vi "Include_when_Saving.vi"(8 "error in (no error)":errorcluster, 11 "AB_Source_Container in":refnum<class "AB_Source_Container.lvclass">) -> (0 "error out":errorcluster, 2 "include":bool, 3 "AB_Source_Container out":refnum<class "AB_Source_Container.lvclass">)   [LabVIEW 2020, in "AB_Source_Container.lvclass"]
uses:
  <vilib>/AppBuilder/AB_Classes/Source/Container/AB_Source_Container.lvclass
  e:/builds/penguin/labview/branches/2020/dev/dist/vi.lib/AppBuilder/AB_Classes/Source/AB_Source.lvclass
  <vilib>/AppBuilder/AB_Classes/Source/Container/AB_Source_Container.lvclass/AB_Source_Container.ctl
  <vilib>/AppBuilder/AB_Classes/Source/AB_Source.lvclass
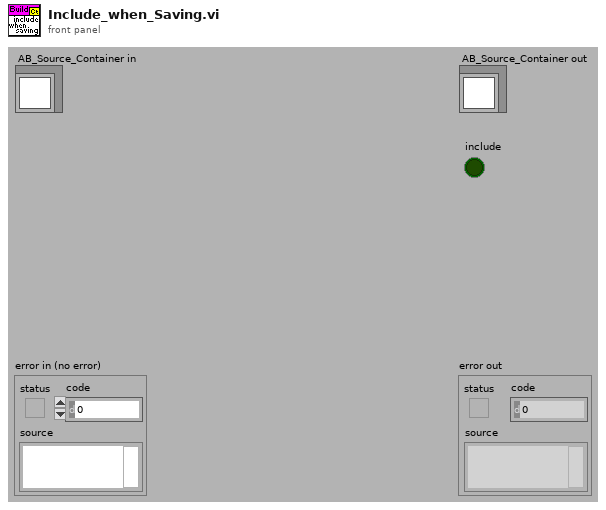
[diagram p1: front panel]
types:
  T1 = typedef "AB_Source.ctl" = cluster{"path":path, "itemID":string, "parentIndex":i32, "sourceInclusion":T2, "destinationIndex":i32, "properties":T3[], "newName":string, "lvfile":bool, "valid":bool, "eng_inBuild":bool, "eng_isNonVILink":bool, "Amalgamation":bool, "Amalgamation Piece":bool, "eng_delimitedName":string, "preventRename":bool}
  T2 = typedef "AB_Source_Inclusion.ctl" = enum16{"IncludeIfReferenced", "Include", "Exclude", "TopLevel"}
  T3 = typedef "AB_Source_Properties.ctl" = cluster{"sourcePropertyType":T4, "value":variant}
  T4 = typedef "AB_Source_Property_Type.ctl" = enum16{"Remove block diagram", "Remove front panel", "Password", "Window has title bar", "Show menu bar", "Show vertical scroll bar", "Show horizontal scroll bar", "Show toolbar", "Show Abort button", "Show fp when called", "Window behavior", "Allow user to close window", "Window run-time position", "Run when opened", "Allow debugging", "Auto error handling", "Generate guard code", "Use stack variables", "Expression folding", "Integer only", "Inline subVI"}
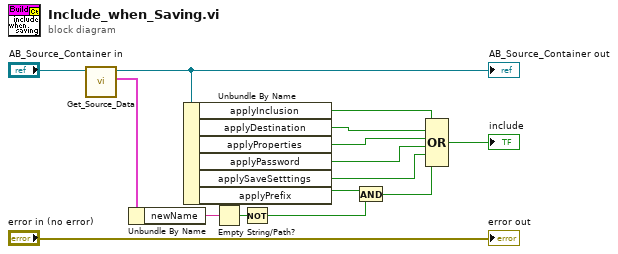
[diagram p0: block diagram]
diagram:
  n1 = call <vilib>:"Get_Source_Data.vi"("Class in"="AB_Source_Container in") -> ("data"=w2:T1, "Class out"=w3:refnum<class "AB_Source_Container.lvclass">)  [unwired: 8 in, 1 out]
  "AB_Source_Container out" <- w3
  n2 = Unbundle By Name(w2) -> ("newName"=w1:string)
  n3 = Unbundle By Name(w3) -> ("applyInclusion"=w14:bool, "applyDestination"=w13:bool, "applyProperties"=w11:bool, "applyPassword"=w12:bool, "applySaveSetttings"=w9:bool, "applyPrefix"=w8:bool)
  n4 = Empty String/Path?(string/path=w1) -> (empty?=w7:bool)
  n5 = Not(x=w7) -> (.not. x?=w6:bool)
  n6 = And(x=w8, y=w6) -> (x .and. y?=w5:bool)
  n7 = Compound Arithmetic op=OR(w14, w13, w11, w12, w9, w5) -> (→"include":bool)
  "error out" <- "error in (no error)"
